vi "tagged refs.vi"(1 "Tags":string[](array[string]), 2 "VI":refnum<vi>) -> (0 "tagged controls":refnum<vi>[](array[refnum]))   [LabVIEW 2012]
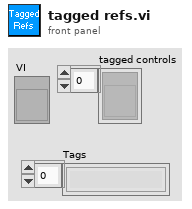
[diagram p1: front panel]
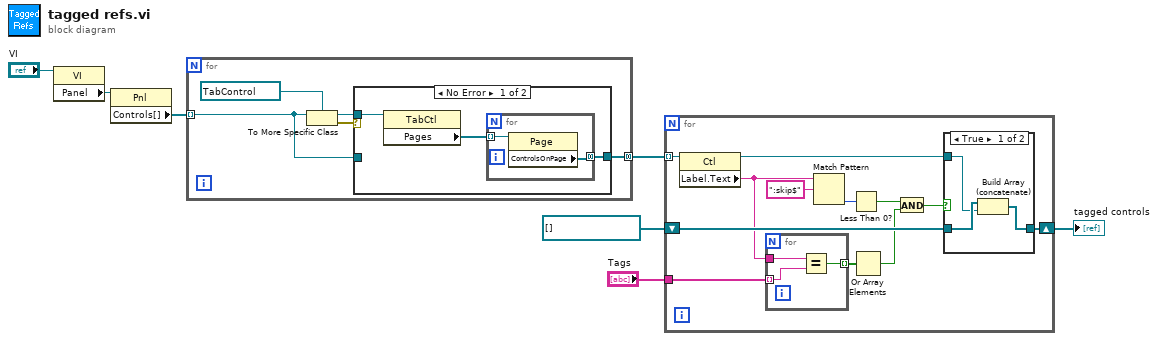
[diagram p0: block diagram]
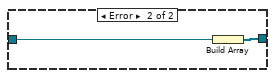
[diagram p3: hidden frame]
diagram:
  n1 = property class="VI"(reference="VI") -> ("Panel"=w7:refnum<vi>)  [unwired: 1 in, 2 out]
  n2 = property class="Pnl"(reference=w7) -> ("Controls[]"=w6:refnum<vi>[])  [unwired: 1 in, 2 out]
  n3 = for {
    tunnel: w6 -> [w9] mode=indexing
    tunnel: [w8] -> w4 mode=concatenating
    n4 = To More Specific Class(target class=refnum<vi> refnum ("reference"), reference=w9) -> (specific class reference=w11:refnum<vi>, error out=w10:errorcluster)  [unwired: 1 in]
    n5 = case shown="No Error" w10 {
      tunnel: w11 -> [w15 _]
      tunnel: [w13 w19] -> w8
      tunnel: w9 -> [_ w18]
      frame No Error {
        n6 = property on="Property Node" class="TabCtl"(reference=w15) -> ("Pages"=w14:refnum<vi>[])  [unwired: 1 in, 2 out]
        n7 = for {
          tunnel: w14 -> [w17] mode=indexing
          tunnel: [w16] -> w13 mode=concatenating
          n8 = property class="Page"(reference=w17) -> ("ControlsOnPage"=w16:refnum<vi>[])  [unwired: 1 in, 2 out]
        }
      }
      frame Error {
        n9 = Build Array(w18) -> (w19:refnum<vi>[])
      }
    }
  }
  n10 = for {
    tunnel: w4 -> [w31] mode=indexing
    shift-right: [w28] -> w2
    shift-left: refnum<vi>[] [] ("all controls") -> [w30]
    tunnel: "Tags" -> [w25]
    n11 = property class="Ctl"(reference=w31) -> (reference out=w29:refnum<vi>, "Label.Text"=w24:string)  [unwired: 1 in, 1 out]
    n12 = for {
      tunnel: w25 -> [w33] mode=indexing
      tunnel: w24 -> [w34]
      tunnel: [w32] -> w23 mode=indexing
      n13 = Equal?(x=w34, y=w33) -> (x = y?=w32:bool)
    }
    n14 = Match Pattern(string=w24, regular expression=":skip$") -> (offset past match=w26:i32)  [unwired: 1 in, 3 out]
    n15 = Less Than 0?(x=w26) -> (x < 0?=w22:bool)
    n16 = Or Array Elements(Boolean array=w23) -> (logical OR=w20:bool)
    n17 = And(x=w22, y=w20) -> (x .and. y?=w21:bool)
    n18 = case shown="True" w21 {
      tunnel: w30 -> [w37 w38]
      tunnel: w29 -> [w36 _]
      tunnel: [w35 w38] -> w28
      frame True {
        n19 = Build Array (concatenate)(w37, w36) -> (w35:refnum<vi>[])
      }
      frame False {
      }
    }
  }
  "tagged controls" <- w2
